vi "PicoScope4000aExampleAWG.vi"() -> ()   [LabVIEW 2010]
uses:
  Program Files/Pico Technology/SDK/lib/ps4000a.dll
panel:
  in  "General AWG Settings":T1={"Peak-to-Peak Voltage (microvolts)"=2000000, "Offset Voltage (microvolts)"=0, "Wave Type"=0, "Sweep Type"=0, "Shots"=0, "Sweeps"=0, "Trigger Type"=0, "Trigger Source"=0, "Ext. Threshold (ADC count)"=0, "White Noise/PRBS"=0} {"White Noise/PRBS" items=["Normal", "White Noise", "PRBS"]; "Trigger Source" items=["None", "Scope Trigger", "Aux. In", "Ext. In", "Software Trigger"]; "Trigger Type" items=["Rising", "Falling", "Gate High", "Gate Low"]; "Sweep Type" items=["Up", "Down", "Up-Down", "Down-Up"]; "Wave Type" items=["Sine", "Square", "Triangle", "Ramp Up", "Ramp Down", "Sinc", "Gaussian", "Half Sine", "DC", "Arbitrary"]}
  out "Unit Info":T2
  out "USB 3.0 on non-USB 3.0 port":bool=TRUE
  out "USB powered":bool=TRUE
  in  "Arbitrary Waveform Settings":T3={"Arbirary waveform file path"=path "", "Start Delta Phase"=1000, "Index Mode"=0, "Stop Delta Phase"=1000, "Delta Phase Increment"=0, "Dwell Count"=0} {"Index Mode" items=["Single", "Dual", "Quad"]}
  in  "Serial Number":string
  in  "Open using Serial Number":bool
  in  "Stop S/W \nTrigger":bool
  in  "Apply Settings":bool
  in  "Stop VI":bool
  in  "Software \nTrigger":bool
  out "Arbitrary\nWaveform Graph":i16[](graph)
  in  "Standard Waveform Settings":T4={"Start Frequency (Hz)"=1000.0, "Stop Frequency (Hz)"=1000.0, "Increment (Hz)"=0.0, "Dwell Time (seconds)"=0.0} {"Start Frequency (Hz)" min=1 max=1000000}
  # "If Software trigger is selected, press the 'Stop S/W Trigger'\nbutton prior to selecting 'Apply Settings' or 'Stop VI'."
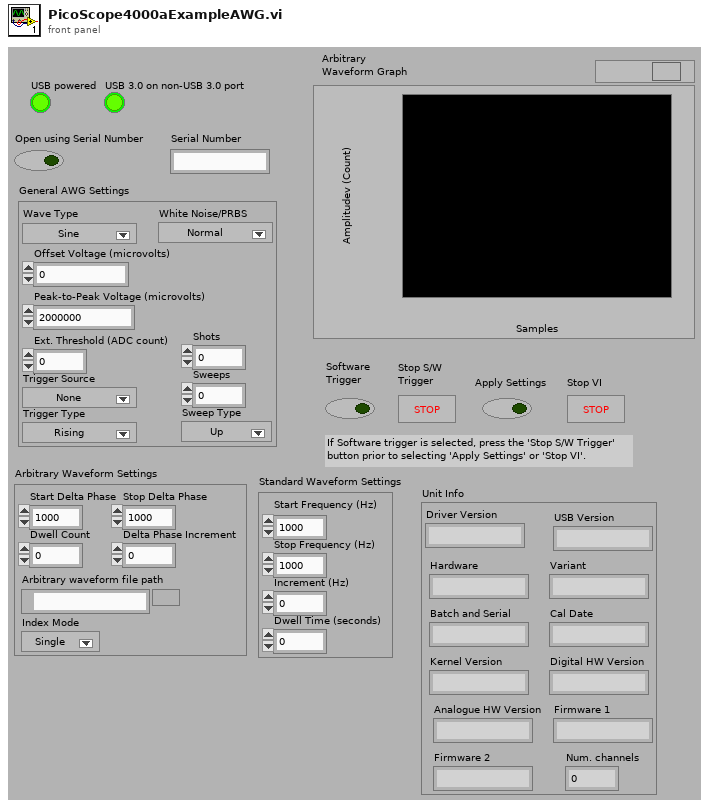
[diagram p1: front panel]
types:
  T1 = cluster{"Peak-to-Peak Voltage (microvolts)":u32, "Offset Voltage (microvolts)":i32, "Wave Type":u32, "Sweep Type":u32, "Shots":u32, "Sweeps":u32, "Trigger Type":u32, "Trigger Source":u32, "Ext. Threshold (ADC count)":i16, "White Noise/PRBS":u32}
  T2 = cluster{"Driver Version":string, "USB Version":string, "Hardware":string, "Variant":string, "Batch and Serial":string, "Cal Date":string, "Kernel Version":string, "Digital HW Version":string, "Analogue HW Version":string, "Firmware 1":string, "Firmware 2":string, "Num. channels":i16}
  T3 = cluster{"Arbirary waveform file path":path, "Start Delta Phase":u32, "Index Mode":i32, "Stop Delta Phase":u32, "Delta Phase Increment":u32, "Dwell Count":u32}
  T4 = cluster{"Start Frequency (Hz)":sgl, "Stop Frequency (Hz)":sgl, "Increment (Hz)":sgl, "Dwell Time (seconds)":sgl}
  T5 = cluster{"status":bool, "code":u32, "source":string}
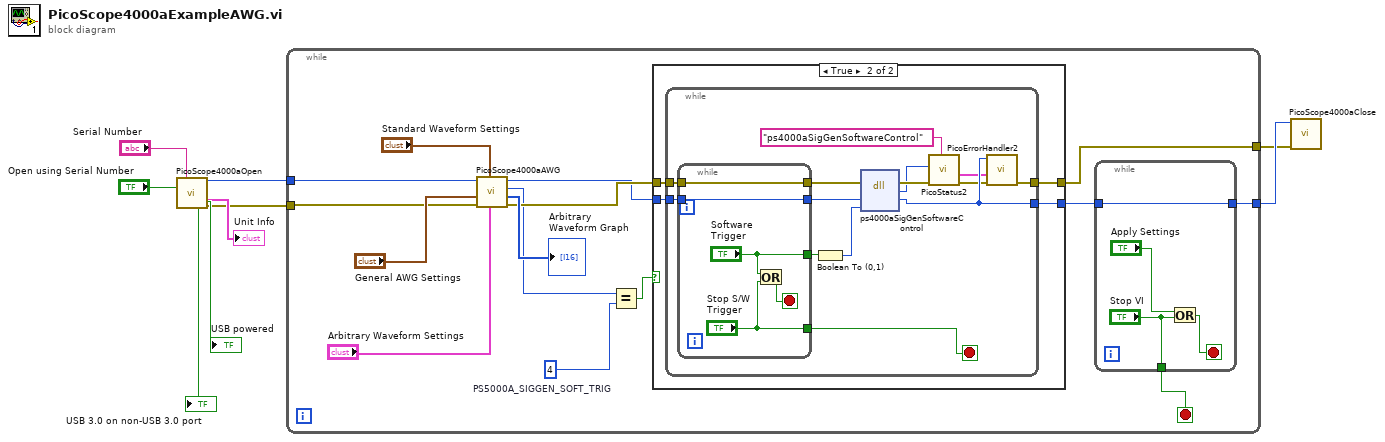
[diagram p0: block diagram]
diagram:
  n1 = call "PicoScope4000aOpen.vi"("Serial Number"="Serial Number", "Use Serial Number"="Open using Serial Number") -> ("handle"=w1:i16, "Unit Info"=→"Unit Info":T2, "USB powered"=→"USB powered":bool, "USB 3.0 on non-USB 3.0 port"=→"USB 3.0 on non-USB 3.0 port":bool, "error out"=w2:errorcluster)  [unwired: 6 in, 3 out]
  n2 = while {
    tunnel: w1 -> [w13]
    tunnel: w2 -> [w14]
    tunnel: [w22] -> w4
    tunnel: [w16] -> w3
    stop <- w21 stop-if-true
    w24 = 4  # PS5000A_SIGGEN_SOFT_TRIG
    n3 = call "PicoScope4000aAWG.vi"("Arbitrary Waveform Settings"="Arbitrary Waveform Settings", "Standard Waveform Settings"="Standard Waveform Settings", "error in"=w14, "General AWG Settings"="General AWG Settings", "Handle In"=w13) -> ("error out"=w12:errorcluster, "Arbitrary\nWaveform Graph"=→"Arbitrary\nWaveform Graph":i16[], "Trigger Source Out"=w10:u32, "Handle Out"=w11:i16)  [unwired: 3 in]
    n4 = Equal?(x=w10, y=w24) -> (x = y?=w23:bool)
    n5 = case shown="True" w23 {
      tunnel: w12 -> [w29 w34]
      tunnel: [w30 w32] -> w17
      tunnel: w11 -> [w30 w33]
      tunnel: [w29 w31] -> w16
      frame False {
      }
      frame True {
        n6 = while {
          tunnel: w34 -> [w47]
          tunnel: w33 -> [w46]
          tunnel: [w38] -> w32
          tunnel: [w35] -> w31
          stop <- w42 stop-if-true
          n7 = while {
            tunnel: [w53] -> w48
            tunnel: w47 -> [w53]
            tunnel: ["Software \nTrigger"] -> w44
            tunnel: w46 -> [w52]
            tunnel: [w52] -> w45
            tunnel: ["Stop S/W \nTrigger"] -> w42
            stop <- w49 stop-if-true
            n8 = Or(x="Software \nTrigger", y="Stop S/W \nTrigger") -> (x .or. y?=w49:bool)
          }
          n9 = Boolean To (0,1)(Boolean=w44) -> (0, 1=w43:i16)
          n10 = dll-call lib="/Program Files/Pico Technology/SDK/lib/ps4000A.dll" fn="ps4000aSigGenSoftwareControl"(error in=w48, "handle"=w45, "state"=w43) -> (error out=w40:errorcluster, "PICO_STATUS"=w39:u32, "handle"=w38:i16)  [unwired: 3 in, 1 out]
          n11 = call "PicoStatus2.vi"("PICO source"="ps4000aSigGenSoftwareControl" ("source"), "Error in"=w40, "PICO STATUS"=w39) -> ("error out"=w37:errorcluster, "PICO_STATUS out"=w36:T5)  [unwired: 5 in]
          n12 = call "PicoErrorHandler2.vi"("error in (no error)"=w37, "PICO_STATUS in"=w36, "handle In"=w38) -> ("error out"=w35:errorcluster)  [unwired: 8 in]
        }
      }
    }
    n13 = while {
      tunnel: ["Stop VI"] -> w21
      tunnel: [w28] -> w22
      tunnel: w17 -> [w28]
      stop <- w27 stop-if-true
      n14 = Or(x="Apply Settings", y="Stop VI") -> (x .or. y?=w27:bool)
    }
  }
  n15 = call "PicoScope4000aClose.vi"("error in (no error)"=w3, "handle in"=w4) -> ()  [unwired: 7 in, 2 out]
